vi "HFRR ADV v06 new software.vi"() -> ()   [LabVIEW 2025] (continued)
                    n2725 = Concatenate Strings(w3588, ".txt" ("string")) -> (w3589:string)
                  }
                }
                n2726 = local read "Test Date"() -> (w3580:string)
                n2727 = local read "String 45"() -> (w3494:string)
                n2728 = local read "String 31"() -> (w3579:string)
                n2729 = local read "String 32"() -> (w3578:string)
                n2730 = local read "TITTLE"() -> (w3502:string)
                n2731 = Number To Fractional String(number=w3549, width (-)=i16 6, precision (6)=i16 2) -> (F-format string=w3548:string)  [unwired: 1 in]
                n2732 = Number To Fractional String(number=w3563, width (-)=i16 6, precision (6)=i16 2) -> (F-format string=w3569:string)  [unwired: 1 in]
                n2733 = Number To Fractional String(number=w3564, width (-)=i16 6, precision (6)=i16 2) -> (F-format string=w3562:string)  [unwired: 1 in]
                n2734 = Number To Fractional String(number=w3568, width (-)=i16 6, precision (6)=i16 2) -> (F-format string=w3567:string)  [unwired: 1 in]
                n2735 = Number To Fractional String(number=w3560, width (-)=i16 6, precision (6)=i16 2) -> (F-format string=w3558:string)  [unwired: 1 in]
                n2736 = Number To Fractional String(number=w3561, width (-)=i16 6, precision (6)=i16 2) -> (F-format string=w3559:string)  [unwired: 1 in]
                n2737 = Number To Fractional String(number=w3572, width (-)=i16 6, precision (6)=i16 2) -> (F-format string=w3573:string)  [unwired: 1 in]
                n2738 = Number To Fractional String(number=w3576, precision (6)=i16 2) -> (F-format string=w3577:string)  [unwired: 2 in]
                n2739 = local read "s.NO"() -> (w3496:string)
                n2740 = Concatenate Strings("=" ("string"), w3502) -> (w3501:string)
                n2741 = Concatenate Strings("S.No," ("string"), "                                       Parameters" ("string")) -> (w3507:string)
                n2742 = Concatenate Strings(w3574, w3533, w3548, w3574, w3530, w3569, w3574, w3529, w3562, w3574, w3525, w3567, w3574, w3523, w3558, w3574, w3520, w3559, w3574, w3517, w3573, w3574, w3514, w3577) -> (w3536:string)
                n2743 = Concatenate Strings(w3506, "," ("string"), w3494, w3496, w3495, w3578, w3581, w3495, w3579, w3580, w3506) -> (w3504:string)
                n2744 = local read "Tested by"() -> (w3510:string)
                n2745 = local read "String 33"() -> (w3511:string)
                n2746 = Concatenate Strings("," ("string"), "                                                                             " ("string")) -> (w3499:string)
                n2747 = Concatenate Strings(w3501, w3497, w3504, w3497, w3507, w3536, w3497, w3499, w3511, w3510) -> (→"export":string)
                n2748 = String To Path(string=w3538) -> (path=w3545:path)
                n2749 = local read "export"() -> (w3540:string)
                n2750 = call <vilib>:"Write Characters To File.vi"("append to file? (new file:F)"=FALSE, "character string"=w3540, "file path (dialog if empty)"=w3545) -> ()  [unwired: 2 in, 1 out]
              }
            }
          }
          frame Enabled {
          }
        }
        n2751 = case shown="True" "OK Button 17" {
          frame False {
          }
          frame True {
            (unwired) 0  # existing file
            w3798 = "Choose a datalog file to open"  # prompt
            n2752 = local write "OK Button 17"(FALSE ("OK Button 17")) -> ()
            n2753 = local read "String"() -> (w3793:string)
            n2754 = String To Path(string=w3793) -> (path=w3794:path)
            n2755 = File Dialog(6:"*.duf" ("pattern"), 7:w3798, 11:w3794) -> (0:w3785:errorcluster, 3:w3804:path)  [unwired: 4 in, 2 out]
            n2756 = Unbundle(w3785) -> ()  [unwired: 3 out]
            n2757 = Open/Create/Replace File "Open File"(file path (use dialog)=w3804) -> (refnum out=w3796:refnum<file>)  [unwired: 5 in, 2 out]
            n2758 = Strip Path(path=w3804) -> (name=w3802:string)  [unwired: 1 out]
            n2759 = Path To String(path=w3804) -> (string=w3787:string)
            n2760 = while {
              tunnel: w3796 -> [w3808]
              i -> [w3805]
              stop <- w3806 continue-if-true
              (unwired) TRUE ("line mode (F)")
              n2761 = Read from Text File "Read File"(file (use dialog)=w3808) -> (text=w3807:string)  [unwired: 3 in, 3 out]
              n2762 = local write "Numeric 16"(w3805) -> ()
              n2763 = String Length(string=w3807) -> (length=w3810:i32)
              n2764 = Greater?(x=w3810, y=1) -> (0:w3806:bool)
            }
            n2765 = local write "String 29"(w3787) -> ()
            n2766 = Search and Replace String(input string=w3787, search string=".duf", replace string=".dgf" ("replace string (\"\")")) -> (result string=→"String Indicator 4":string)  [unwired: 5 in, 3 out]
            n2767 = Match Pattern(string=w3802, regular expression=".dwm") -> (before substring=w3786:string)  [unwired: 1 in, 3 out]
            "String Indicator" <- w3786
            n2768 = Match Pattern(string=w3787, regular expression=".dwm" ("substring (\"\")")) -> (before substring=w3788:string)  [unwired: 1 in, 3 out]
            "String Indicator 3" <- w3788
            n2769 = local write "TITTLE 2"(w3786) -> ()
            n2770 = String To Path(string=w3788) -> (path=w3795:path)
            "path" <- w3795
            n2771 = call <vilib>:"Read Characters From File.vi"("file path (dialog if empty)"=w3795, "start of read offset (chars.:0)"=60 ("start of read offset (chars.: 0)")) -> ("character string"=→"String Indicator 2":string)  [unwired: 4 in, 3 out]
          }
        }
        n2772 = call <vilib>:"Query Available Printers.vi"() -> ("system configured printers"=w3487:string[])  [unwired: 9 in, 2 out]
        "System Configured Printers 2" <- w3487
        n2773 = local read "OK Button 16"() -> (w3484:bool)
        n2774 = case shown="True" "OK Button 16" {
          frame False {
          }
          frame True {
            n2775 = stacked-sequence {
              frame #0 {
                n2776 = local read "Numeric 16"() -> (w3812:i32)
                n2777 = local write "Numeric 10"(w3812) -> ()
              }
              frame #1 {
                n2778 = local read "S.NO"() -> (→"s.NO":string)
                n2779 = local read "String 29"() -> (w3816:string)
                n2780 = String To Path(string=w3816) -> (path=w3815:path)
                n2781 = Open/Create/Replace File "Open File"(file path (use dialog)=w3815) -> (refnum out=w3817:refnum<file>)  [unwired: 5 in, 2 out]
                n2782 = for {
                  N: 16 -> [_]
                  tunnel: w3817 -> [w3824]
                  i -> [w3820]
                  (unwired) TRUE ("line mode (F)")
                  n2783 = Read from Text File "Read File"(file (use dialog)=w3824) -> (text=w3818:string)  [unwired: 3 in, 3 out]
                  n2784 = Match Pattern(string=w3818, regular expression="(") -> (after substring=w3823:string)  [unwired: 1 in, 3 out]
                  n2785 = Match Pattern(string=w3823, regular expression=")") -> (before substring=w3819:string)  [unwired: 1 in, 3 out]
                  n2786 = case shown="1" w3820 {
                    tunnel: w3819 -> [w3825 w3826 _ _ w3827 w3828 w3829 w3831 w3833 w3835 w3837 w3839 w3841 w3843 _]
                    tunnel: w3818 -> [_ _ _ _ _ _ _ _ _ _ _ _ _ _ _]
                    frame 0 {
                      "TITTLE" <- w3825
                    }
                    frame 1 {
                      "Sample ID" <- w3826
                    }
                    frame 2 {
                    }
                    frame 3 {
                    }
                    frame 4 {
                      "Test Date" <- w3827
                    }
                    frame 5 {
                      "Tested by" <- w3828
                    }
                    frame 6 {
                      n2787 = Fract/Exp String To Number(string=w3829) -> (number=→"Humidity before test 2":dbl)  [unwired: 3 in, 1 out]
                    }
                    frame 7 {
                      n2788 = Fract/Exp String To Number(string=w3831) -> (number=→"Temperature before test 2":dbl)  [unwired: 3 in, 1 out]
                    }
                    frame 8 {
                      n2789 = Fract/Exp String To Number(string=w3833) -> (number=→"Humidity after test 2":dbl)  [unwired: 3 in, 1 out]
                    }
                    frame 9 {
                      n2790 = Fract/Exp String To Number(string=w3835) -> (number=→"Temperature after test 2":dbl)  [unwired: 3 in, 1 out]
                    }
                    frame 10 {
                      n2791 = Fract/Exp String To Number(string=w3837) -> (number=→"MWSD 2":dbl)  [unwired: 3 in, 1 out]
                    }
                    frame 11 {
                      n2792 = Fract/Exp String To Number(string=w3839) -> (number=→"AVP 2":dbl)  [unwired: 3 in, 1 out]
                    }
                    frame 12 {
                      n2793 = Fract/Exp String To Number(string=w3841) -> (number=→"HCF 2":dbl)  [unwired: 3 in, 1 out]
                    }
                    frame 13 {
                      n2794 = Fract/Exp String To Number(string=w3843) -> (number=→"WS1.4 2":dbl)  [unwired: 3 in, 1 out]
                    }
                    frame 14, Default {
                    }
                  }
                }
              }
              frame #2 {
              }
            }
            n2795 = local write "OK Button 16"(FALSE ("OK Button 13")) -> ()
          }
        }
        n2796 = Index Array(array=w3487, index="Select Printer 3") -> (element=w3489:string)
        "Selected Printer" <- w3489
        n2797 = case shown="True" w3484 {
          frame False {
          }
          frame True {
            n2798 = flat-sequence {
              frame #0 {
              }
              frame #1 {
                n2799 = Wait (ms)(milliseconds to wait=u32 100) -> ()  [unwired: 1 out]
              }
              frame #2 {
                n2800 = local write "OK Button 16"(FALSE ("Print 3")) -> ()
              }
            }
          }
        }
        n2801 = case shown="True" "Print" {
          tunnel: w3489 -> [_ w3781]
          frame False {
          }
          frame True {
            (unwired) i16 6 ("width (-)")
            (unwired) "TESTED BY : "
            (unwired) "TESTED DATE :"
            (unwired) "SAMPLE ID : "
            (unwired) "SAMPLE DESIGN : "
            w3739 = "\r"
            w3756 = "\r"
            # "add image"
            n2802 = local read "Sample ID"() -> (w3729:string)
            n2803 = local read "Tested by"() -> (w3732:string)
            n2804 = local read "String 34"() -> (w3719:string)
            n2805 = local read "String 45"() -> (w3699:string)
            n2806 = local read "String 35"() -> (w3714:string)
            n2807 = local read "String 37"() -> (w3712:string)
            n2808 = local read "String 32"() -> (w3734:string)
            n2809 = local read "String 36"() -> (w3709:string)
            n2810 = local read "String 31"() -> (w3733:string)
            n2811 = local read "Test Date"() -> (w3730:string)
            n2812 = local read "String 33"() -> (w3735:string)
            n2813 = local read "String 38"() -> (w3705:string)
            n2814 = local read "String 39"() -> (w3702:string)
            n2815 = local write "Print"(FALSE ("Print FF")) -> ()
            n2816 = local read "S 39"() -> (w3717:string)
            n2817 = local read "S 38"() -> (w3724:string)
            n2818 = local read "Temperature before test 2"() -> (w3755:dbl)
            n2819 = local read "Temperature after test 2"() -> (w3745:dbl)
            n2820 = local read "Humidity before test 2"() -> (w3770:dbl)
            n2821 = local read "Humidity after test 2"() -> (w3754:dbl)
            n2822 = local read "MWSD 2"() -> (w3759:dbl)
            n2823 = local read "WS1.4 2"() -> (w3737:dbl)
            n2824 = Concatenate Strings("2)" ("string"), w3719) -> (w3720:string)
            n2825 = Concatenate Strings("3)" ("string"), w3717) -> (w3718:string)
            n2826 = Concatenate Strings("1)" ("string"), w3724) -> (w3723:string)
            n2827 = Concatenate Strings("4)" ("string"), w3714) -> (w3715:string)
            n2828 = Concatenate Strings("5)" ("string"), w3712) -> (w3711:string)
            n2829 = Concatenate Strings("6)" ("string"), w3709) -> (w3708:string)
            n2830 = Concatenate Strings("7)" ("string"), w3705) -> (w3706:string)
            n2831 = Concatenate Strings("8)" ("string"), w3702) -> (w3703:string)
            n2832 = local read "HCF 2"() -> (w3741:dbl)
            n2833 = local read "AVP 2"() -> (w3758:dbl)
            n2834 = local read "s.NO"() -> (w3700:string)
            n2835 = call <vilib>:"New Report.vi"("report type"=enum16{"Standard Report", "HTML"}."Standard Report") -> ("report out"=w3779:refnum<class "NI_report.lvclass">, "error out"=w3778:errorcluster)  [unwired: 13 in]
            n2836 = local read "TITTLE"() -> (w3731:string)
            n2837 = Concatenate Strings(w3756, w3699, w3700, w3756, w3734, w3729, w3756, w3733, w3730, w3756, w3735, w3732, w3756) -> (w3749:string)
            "test by" <- w3749
            n2838 = Number To Fractional String(number=w3755, width (-)=i16 6, precision (6)=i16 2) -> (F-format string=w3744:string)  [unwired: 1 in]
            n2839 = Number To Fractional String(number=w3754, width (-)=i16 6, precision (6)=i16 2) -> (F-format string=w3757:string)  [unwired: 1 in]
            n2840 = Number To Fractional String(number=w3770, width (-)=i16 6, precision (6)=i16 2) -> (F-format string=w3775:string)  [unwired: 1 in]
            n2841 = Number To Fractional String(number=w3759, width (-)=i16 6, precision (6)=i16 2) -> (F-format string=w3761:string)  [unwired: 1 in]
            n2842 = Number To Fractional String(number=w3745, width (-)=i16 6, precision (6)=i16 2) -> (F-format string=w3746:string)  [unwired: 1 in]
            n2843 = Number To Fractional String(number=w3758, width (-)=i16 6, precision (6)=i16 2) -> (F-format string=w3760:string)  [unwired: 1 in]
            n2844 = Number To Fractional String(number=w3741, width (-)=i16 6, precision (6)=i16 2) -> (F-format string=w3740:string)  [unwired: 1 in]
            n2845 = Number To Fractional String(number=w3737, precision (6)=i16 2) -> (F-format string=w3736:string)  [unwired: 2 in]
            n2846 = call-dynamic "Set Report Header Text.vi"("report in"=w3779, "center header text"=w3731, "error in (no error)"=w3778) -> ("report out"=w3750:refnum<class "NI_report.lvclass">, "error out"=w3751:errorcluster)  [unwired: 11 in]
            n2847 = Concatenate Strings(w3739, w3723, w3775, w3739, w3720, w3744, w3739, w3718, w3757, w3739, w3715, w3746, w3739, w3711, w3761, w3739, w3708, w3760, w3739, w3706, w3740, w3739, w3703, w3736) -> (w3727:string)
            "export 2" <- w3727
            n2848 = call-poly <vilib>:"Append Report Text.vi"("report in"=w3750, "text"=w3749, "error in (no error)"=w3751) -> ("report out"=w3753:refnum<class "NI_report.lvclass">, "error out"=w3752:errorcluster)  [unwired: 9 in, 2 out]
            n2849 = local read "test by"() -> (w3726:string)
            n2850 = local read "TITTLE"() -> (w3728:string)
            n2851 = call-poly <vilib>:"Append Report Text.vi"("report in"=w3753, "error in (no error)"=w3752) -> ("report out"=w3774:refnum<class "NI_report.lvclass">, "error out"=w3772:errorcluster)  [unwired: 10 in, 2 out]
            n2852 = Concatenate Strings(w3728, w3727, w3726) -> (→"output":string)
            n2853 = call-poly <vilib>:"Append Report Text.vi"("report in"=w3774, "text"=w3727, "error in (no error)"=w3772) -> ("report out"=w3773:refnum<class "NI_report.lvclass">, "error out"=w3771:errorcluster)  [unwired: 9 in, 2 out]
            n2854 = call-dynamic "Print Report.vi"("report in"=w3773, "printer name (default)"=w3781, "error in (no error)"=w3771) -> ("report out"=w3783:refnum<class "NI_report.lvclass">, "error out"=w3784:errorcluster)  [unwired: 11 in]
            n2855 = call-dynamic "Dispose Report.vi"("report in"=w3783, "error in (no error)"=w3784) -> ()  [unwired: 13 in, 1 out]
          }
        }
        n2856 = case shown="True" "Print 2" {
          frame False {
          }
          frame True {
            n2857 = flat-sequence {
              frame #0 {
                n2858 = local read "s.NO"() -> (→"s.NO 2":string)
                n2859 = Wait (ms)(milliseconds to wait=u32 20) -> ()  [unwired: 1 out]
                n2860 = local read "Sample ID  3"() -> (→"Sample ID  6":string)
                n2861 = local read "Sample ID  4"() -> (→"Sample ID  7":string)
                n2862 = local read "Sample ID"() -> (→"Sample ID  2":string)
                n2863 = local read "Tested by"() -> (→"Tested by 2":string)
                n2864 = local read "Test Date"() -> (→"Test Date 2":string)
                n2865 = local read "Humidity after test 3"() -> (→"Humidity after test 4":dbl)
                n2866 = local read "Ref A Test Date :"() -> (→"TITTLE 4":string)
                n2867 = local read "Temperature before test 3"() -> (w3606:dbl)
                n2868 = local read "Temperature before test 3"() -> (→"Temperature after test 5":dbl)
                n2869 = local read "Temperature after test 3"() -> (→"Temperature after test 4":dbl)
                n2870 = local read "Humidity before test 3"() -> (→"Humidity before test 4":dbl)
                n2871 = local write "Temperature before test 3"(w3606) -> ()
                n2872 = local read "image data"() -> (w3597:T11)
                n2873 = String To Path(string="C:\\LAB-IQ\\im\\Temp_resized.jpg") -> (path=w3598:path)
                "path 2" <- w3598
                n2874 = call <vilib>:"Write JPEG File.vi"("image data"=w3597, "path to JPEG file"=w3598) -> ()  [unwired: 8 in, 2 out]
                "Ref A Test Date :" <- "Ref A Test Date :"
                "Ref B Test Date :" <- "Ref B Test Date :"
                "Ref B Scar Value :" <- "Ref B Scar Value :"
                "Ref A Scar Value :" <- "Ref A Scar Value :"
              }
              frame #1 {
                (unwired) HTML_Report_Image_Alignment."MIDDLE" ("alignment (default)")
                w3634 = u16 0 items=["portrait", "landscape"] ("orientation (portrait)")
                (unwired) HTML_Report_Image_Alignment."ABSMIDDLE" ("alignment (default)")
                (unwired) "TESTED BY : "
                (unwired) "TESTED DATE :"
                (unwired) "SAMPLE ID : "
                (unwired) "SAMPLE DESIGN : "
                w3667 = "\r"
                # "add image"
                n2875 = Wait (ms)(milliseconds to wait=u32 20) -> ()  [unwired: 1 out]
                n2876 = local read "Sample ID  2"() -> (w3660:string)
                n2877 = local read "Wear Scar X"() -> (w3632:dbl)
                "Length ( microns ) 2" <- w3632
                n2878 = local read "Wear Scar Y"() -> (w3631:dbl)
                "Wear Scar Y ( microns ) :" <- w3631
                n2879 = local read "Test Date 2"() -> (w3661:string)
                n2880 = local read "Tested by 2"() -> (w3662:string)
                n2881 = local read "String 46"() -> (w3658:string)
                n2882 = local read "String 48"() -> (w3664:string)
                n2883 = local read "String 47"() -> (w3663:string)
                n2884 = local read "String 49"() -> (w3665:string)
                n2885 = local read "String 10"() -> (w3618:string)
                n2886 = local read "s.NO 2"() -> (w3659:string)
                n2887 = Add(x=w3632, y=w3631) -> (x+y=w3630:dbl)
                n2888 = call <vilib>:"New Report.vi"("report type"=enum16{"Standard Report", "HTML"}."HTML") -> ("report out"=w3638:refnum<class "NI_report.lvclass">, "error out"=w3636:errorcluster)  [unwired: 13 in]
                n2889 = Concatenate Strings(w3667, w3658, w3659, w3667, w3664, w3660, w3667, w3663, w3661, w3667, w3665, w3662, w3667) -> (→"test by 2":string)
                n2890 = Concatenate Strings("C:\\LAB-IQ\\Data\\" ("string"), w3618, ".jpg" ("string")) -> ()  [unwired: 1 out]
                n2891 = Divide(x=w3630, y=2.0) -> (x/y=→"Mean Wear ( microns) :":dbl)
                n2892 = call-dynamic "Set Report Orientation.vi"("report in"=w3638, "orientation (portrait)"=w3634, "error in (no error)"=w3636) -> ("report out"=w3637:refnum<class "NI_report.lvclass">, "error out"=w3635:errorcluster)  [unwired: 11 in]
                n2893 = for {
                  N: 5 -> [_]
                  tunnel: w3637 -> [w3688]
                  tunnel: [w3687] -> w3616
                  tunnel: w3635 -> [w3686]
                  tunnel: [w3685] -> w3615
                  n2894 = call-dynamic "Set Report Tab Width.vi"("report in"=w3688, "error in (no error)"=w3686) -> ("report out"=w3687:refnum<class "NI_report.lvclass">, "error out"=w3685:errorcluster)  [unwired: 12 in]
                }
                n2895 = local read "TITTLE"() -> (w3633:string)
                n2896 = call-dynamic "Set Report Header Text.vi"("report in"=w3616, "center header text"=w3633, "error in (no error)"=w3615) -> ("report out"=w3654:refnum<class "NI_report.lvclass">, "error out"=w3653:errorcluster)  [unwired: 11 in]
                n2897 = for {
                  N: 1 -> [_]
                  tunnel: [w3692] -> w3640
                  tunnel: [w3691] -> w3639
                  tunnel: w3654 -> [w3690]
                  tunnel: w3653 -> [w3689]
                  n2898 = call-dynamic "New Report Line.vi"("report in"=w3690, "error in (no error)"=w3689) -> ("report out"=w3692:refnum<class "NI_report.lvclass">, "error out"=w3691:errorcluster)  [unwired: 12 in]
                }
                n2899 = for {
                  N: 2 -> [_]
                  tunnel: [w3684] -> w3646
                  tunnel: [w3683] -> w3645
                  tunnel: w3640 -> [w3682]
                  tunnel: w3639 -> [w3681]
                  n2900 = call-dynamic "New Report Line.vi"("report in"=w3682, "error in (no error)"=w3681) -> ("report out"=w3684:refnum<class "NI_report.lvclass">, "error out"=w3683:errorcluster)  [unwired: 12 in]
                }
                n2901 = for {
                  N: 25 -> [_]
                  tunnel: w3646 -> [w3680]
                  tunnel: w3645 -> [w3678]
                  tunnel: [w3679] -> w3649
                  tunnel: [w3677] -> w3648
                  n2902 = call-dynamic "Set Report Tab Width.vi"("report in"=w3680, "error in (no error)"=w3678) -> ("report out"=w3679:refnum<class "NI_report.lvclass">, "error out"=w3677:errorcluster)  [unwired: 12 in]
                }
                n2903 = control-ref of="Tab Control 9"() -> (w3644:refnum<vi>)
                n2904 = call-dynamic "Append Control Image to Report.vi"("report in"=w3649, "alignment (default)"=HTML_Report_Image_Alignment."ABSMIDDLE", "ctrl reference"=w3644, "error in (no error)"=w3648) -> ("report out"=w3643:refnum<class "NI_report.lvclass">, "error out"=w3642:errorcluster)  [unwired: 8 in, 2 out]
                n2905 = for {
                  N: 3 -> [_]
                  tunnel: [w3676] -> w3627
                  tunnel: [w3675] -> w3626
                  tunnel: w3643 -> [w3674]
                  tunnel: w3642 -> [w3673]
                  n2906 = call-dynamic "New Report Line.vi"("report in"=w3674, "error in (no error)"=w3673) -> ("report out"=w3676:refnum<class "NI_report.lvclass">, "error out"=w3675:errorcluster)  [unwired: 12 in]
                }
                n2907 = for {
                  N: 100 -> [_]
                  tunnel: w3627 -> [w3672]
                  tunnel: w3626 -> [w3670]
                  tunnel: [w3671] -> w3623
                  tunnel: [w3669] -> w3621
                  n2908 = call-dynamic "Set Report Tab Width.vi"("report in"=w3672, "error in (no error)"=w3670) -> ("report out"=w3671:refnum<class "NI_report.lvclass">, "error out"=w3669:errorcluster)  [unwired: 12 in]
                }
                n2909 = String To Path(string="C:\\LAB-IQ\\im\\Temp_resized.jpg") -> (path=w3613:path)
                n2910 = call-poly <vilib>:"Append Image to Report.vi"("report in"=w3623, "path or URL of image"=w3613, "error in (no error)"=w3621) -> ("report out"=w3622:refnum<class "NI_report.lvclass">, "error out"=w3620:errorcluster)  [unwired: 9 in, 2 out]
                n2911 = call-poly <vilib>:"Open HTML Report in Browser.vi"("report in"=w3622, "error in (no error)"=w3620) -> ("report out"=w3657:refnum<class "NI_report.lvclass">, "error out"=w3656:errorcluster)  [unwired: 11 in, 1 out]
                n2912 = call-dynamic "Dispose Report.vi"("report in"=w3657, "error in (no error)"=w3656) -> ()  [unwired: 13 in, 1 out]
              }
              frame #2 {
              }
              frame #3 {
                n2913 = disable-structure shown="Disabled" {
                  frame Disabled {
                    n2914 = local read "String 10"() -> (w3697:string)
                    n2915 = Concatenate Strings("C:\\LAB-IQ-NXT\\Data\\" ("string"), w3697, ".jpg" ("string")) -> (w3695:string)
                    n2916 = String To Path(string=w3695) -> (path=w3694:path)
                    n2917 = Delete(path (use dialog)=w3694) -> ()  [unwired: 4 in, 3 out]
                  }
                  frame Enabled {
                  }
                }
                n2918 = local write "Print 2"(FALSE ("Print")) -> ()
              }
            }
          }
        }
      }
    }
    n2919 = property on="SetTemp" class="DigNum (strict)"("Disabled"=w1640) -> ()  [unwired: 2 in, 2 out]
    n2920 = Multiply(x=w1630, y=w1632) -> (x*y=w1631:dbl)
    n2921 = local read "MWSD"() -> (w1629:dbl)
    n2922 = Add(x=w1631, y=w1629) -> (x+y=→"WS1.4":dbl)
    n2923 = Wait (ms)(milliseconds to wait=u32 50) -> ()  [unwired: 1 out]
    n2924 = Wait (ms)(milliseconds to wait=u32 50) -> ()  [unwired: 1 out]
    n2925 = local read "Quit"() -> (w1628:bool)
  }
  n2926 = VISA Close(VISA resource name=w52, error in (no error)=w51) -> (error out=w49:errorcluster)
  n2927 = call <vilib>:"Clear Errors.vi"("error in (no error)"=w49) -> ()  [unwired: 5 in, 2 out]
  n2928 = VISA Close(VISA resource name=w37, error in (no error)=w36) -> ()  [unwired: 1 out]
  n2929 = while {
    tunnel: [w3856] -> w46
    shift-right: [w3849] -> _
    shift-left: 0.0 -> [w3852]
    shift-right: [w3848] -> _
    shift-left: 0.0 -> [w3851]
    shift-right: [w3847] -> _
    shift-left: 400.0 ("vc_cmd") -> [w3850]
    stop <- w3856 stop-if-true
    # "PID LOGIC"
    n2930 = local read "RUN"() -> (w3854:bool)
    n2931 = local read "Auto Start Test"() -> (w3853:bool)
    n2932 = local read "START TEMP"() -> (w3845:bool)
    n2933 = Or(x=w3854, y=w3853) -> (x .or. y?=w3855:bool)
    n2934 = And(x=w3855, y=w3845) -> (x .and. y?=w3846:bool)
    n2935 = Wait (ms)(milliseconds to wait=u32 20) -> ()  [unwired: 1 out]
    n2936 = case shown="True" w3846 {
      tunnel: [400.0 ("out_vc_cmd") w3876] -> w3847
      tunnel: [w3859 w3878] -> w3848
      tunnel: [w3859 w3877] -> w3849
      tunnel: w3852 -> [_ w3867]
      tunnel: w3851 -> [_ w3866]
      tunnel: w3850 -> [_ w3865]
      frame False {
        w3859 = 0.0 ("error_out")
      }
      frame True {
        n2937 = local read "Set Strk"() -> (w3862:dbl)
        n2938 = local read "LVDT STROKE"() -> (w3860:dbl)
        n2939 = Add(x=w3862, y="Add up Stroke") -> (x+y=w3863:dbl)
        n2940 = formula code="// Zero-Hardcode Explicit Positional-Form PID Engine\n// Inputs: target_stroke, measured_stroke, dt, prev_error, integral_accumulator_in, prev_vc_cmd\n//         kp, ki, kd, max_step_change, max_amplitude, min_amplitude, startup_cmd\n// Outputs: vc_cmd, error_out, out_error, integral_accumulator_out, out_vc_cmd\n\n// 1. Calculate Tracking Error\nfloat current_error = target_stroke - measured_stroke;\nerror_out = current_error;\n\n// 2. Compute Proportional Term\nfloat p_term = kp * current_error;\n\n// 3. Compute Derivative Term\nfloat d_term = 0.0;\nif (dt > 0.0) {\n    d_term = kd * ((current_error - prev_error) / dt);\n}\n\n// 4. Update and Accumulate Integral Term\nfloat current_integral = integral_accumulator_in + (current_error * dt);\nfloat i_term = ki * current_integral;\n\n// 5. Calculate Ideal Target Command\nfloat ideal_command = startup_cmd + p_term + i_term + d_term;\n\n// 6. Anti-Windup Protection (Back-calculation method)\nif (ideal_command > max_amplitude) {\n    float excess = ideal_command - max_amplitude;\n    if (ki > 0.0) {\n        current_integral -= excess / ki;\n    }\n    ideal_command = max_amplitude;\n} else if (ideal_command < min_amplitude) {\n    float excess = ideal_command - min_amplitude;\n    if (ki > 0.0) {\n        current_integral -= excess / ki;\n    }\n    ideal_command = min_amplitude;\n}\n\n// 7. Apply Loop Rate Limiting (Protects voice coil from large voltage steps)\nfloat raw_adjustment = ideal_command - prev_vc_cmd;\n\nif (raw_adjustment > max_step_change) {\n    raw_adjustment = max_step_change;\n} else if (raw_adjustment < -max_step_change) {\n    raw_adjustment = -max_step_change;\n}\n\nfloat next_vc_cmd = prev_vc_cmd + raw_adjustment;\n\n// Final Output Safety Safeguard Clamping\nif (next_vc_cmd > max_amplitude) {\n    next_vc_cmd = max_amplitude;\n} else if (next_vc_cmd < min_amplitude) {\n    next_vc_cmd = min_amplitude;\n}\n\n// 8. Map to Shift Registers for memory persistence\nvc_cmd = next_vc_cmd;\nout_error = current_error;                     \nintegral_accumulator_out = current_integral;  \nout_vc_cmd = next_vc_cmd;"("target_stroke"=w3863, "measured_stroke"=w3860, "dt"="dt", "integral_accumulator_in"=w3866, "prev_error"=w3867, "prev_vc_cmd"=w3865, "kp"="kp", "ki"="ki", "kd"="kd", "max_step_change"="max_step_change", "max_amplitude"="max_amplitude", "min_amplitude"="min_amplitude", "startup_cmd"="startup_cmd") -> ("vc_cmd"=w3882:dbl, "out_error"=w3877:dbl, "integral_accumulator_out"=w3878:dbl, "out_vc_cmd"=w3876:dbl)  [unwired: 1 out]
        "output Vpp" <- w3882
        n2941 = Number To Fractional String(number=w3882, precision (6)=i16 1) -> (F-format string=w3880:string)  [unwired: 2 in]
        n2942 = Concatenate Strings("DAC;" ("string"), w3880) -> (w3864:string)
        n2943 = local write "Command"(w3864) -> ()
        "prev_error" <- w3867
        "integral_accumulator_in" <- w3866
        "prev_vc_cmd" <- w3865
      }
    }
    n2944 = local read "Quit"() -> (w3856:bool)
  }
  n2945 = Or(x=w42, y=w41) -> (x .or. y?=w43:bool)
  n2946 = Or(x=w39, y=w43) -> (x .or. y?=w48:bool)
  n2947 = control-ref of="new picture"() -> ()  [unwired: 1 out]
  n2948 = Or(x=w54, y=w48) -> (x .or. y?=w45:bool)
  n2949 = Or(x=w45, y=w46) -> (x .or. y?=w40:bool)
  n2950 = while {
    tunnel: [w3883] -> w53
    i -> [w3890]
    stop <- w3883 stop-if-true
    n2951 = local read "Quit"() -> (w3883:bool)
    n2952 = Equal To 0?(x=w3890) -> (x = 0?=w3888:bool)
    n2953 = call "Elapsed Time3"("Time Target (s)"=45.0, "Auto Reset"=TRUE) -> ("Time has Elapsed"=w3887:bool)  [unwired: 10 in, 7 out]
    n2954 = Wait (ms)(milliseconds to wait=u32 50) -> ()  [unwired: 1 out]
    n2955 = Or(x=w3887, y=w3888) -> (x .or. y?=w3889:bool)
    n2956 = case shown="True" w3889 {
      frame False {
      }
      frame True {
        n2957 = call <vilib>:"System Exec.vi"("run minimized? (F)"=TRUE, "error in (no error)"="error in (no error)", "command line"="powercfg.exe -change -monitor-timeout-ac 0") -> ("error out"=w3901:errorcluster)  [unwired: 5 in, 3 out]
        n2958 = call <vilib>:"System Exec.vi"("run minimized? (F)"=TRUE, "error in (no error)"=w3901, "command line"="powercfg.exe -change -disk-timeout-ac 0") -> ("error out"=w3900:errorcluster)  [unwired: 5 in, 3 out]
        n2959 = call <vilib>:"System Exec.vi"("run minimized? (F)"=TRUE, "error in (no error)"=w3900, "command line"="powercfg.exe -change -standby-timeout-ac 0") -> ("error out"=w3899:errorcluster)  [unwired: 5 in, 3 out]
        n2960 = call <vilib>:"System Exec.vi"("run minimized? (F)"=TRUE, "error in (no error)"=w3899, "command line"="powercfg.exe -change -hibernate-timeout-ac 0") -> ("error out"=w3898:errorcluster)  [unwired: 5 in, 3 out]
        n2961 = call <vilib>:"Simple Error Handler.vi"("error in (no error)"=w3898) -> ("error out"=w3904:errorcluster)  [unwired: 4 in, 4 out]
        n2962 = call <vilib>:"Clear Errors.vi"("error in (no error)"=w3904) -> ("error out"=→"error out":errorcluster)  [unwired: 5 in, 1 out]
      }
    }
  }
  n2963 = Compound Arithmetic op=OR(w56, w40, w53) -> (w55:bool)
  n2964 = flat-sequence {
    tunnel: w55 -> [_]
    tunnel: [w3906] -> w18
    tunnel: w18 -> [_]
    frame #0 {
      n2965 = call "CLOSE CONNECTION.vi"() -> ("error out"=w3906:errorcluster)  [unwired: 11 in]
    }
    frame #1 {
      n2966 = Quit LabVIEW(quit? (T)=TRUE) -> ()
      n2967 = local write "Quit"(FALSE ("EXIT")) -> ()
    }
  }
  n2968 = property on="Heater Button" class="Bool (strict)"("Visible"=TRUE) -> ()  [unwired: 2 in, 2 out]
  n2969 = disable-structure shown="Disabled" {
    disable-tunnel: _ -> [w3912 _]
    disable-tunnel: _ -> [w3909 _]
    disable-tunnel: _ -> [w3910 _]
    frame Disabled {
      n2970 = disable-structure shown="Disabled" {
        disable-tunnel: [w3919 _] -> w3911
        frame Disabled {
          n2971 = while {
            shift-right: [w3961] -> w3917
            shift-left: errorcluster {"status"=TRUE, "code"=0, "source"="Init"} ("error out") -> [w3926]
            shift-right: [w3960] -> w3916
            shift-left: _ -> [w3927]
            shift-right: [w3959] -> _
            shift-left: "" -> [w3958]
            tunnel: [w3920] -> w3919
            shift-right: ["Set Rh"] -> _
            shift-left: 0.0 ("Set Rh") -> [w3952]
            tunnel: [w3929] -> _
            i -> [w3929]
            stop <- w3920 stop-if-true
            n2972 = flat-sequence {
              tunnel: w3926 -> [w3964]
              tunnel: [w3964] -> w3925
              frame #0 {
                n2973 = Wait (ms)(milliseconds to wait=u32 200) -> ()  [unwired: 1 out]
              }
            }
            n2974 = local read "Com Port 3"() -> (w3928:refnum<visa-resource-name>)
            n2975 = local read "Humidity Str Rec"() -> (w3930:string)
            n2976 = Not Equal?(x="Set Rh", y=w3952) -> (x != y?=w3957:bool)
            n2977 = Number To Decimal String(number="Set Rh") -> (decimal integer string=w3955:string)  [unwired: 1 in]
            n2978 = Not Equal?(x=w3928, y=w3927) -> (x != y?=w3923:bool)
            n2979 = Concatenate Strings("#setPoint00" ("string"), w3955) -> (w3956:string)
            n2980 = case shown="False" w3957 {
              tunnel: w3956 -> [_ w3976]
              frame False {
                n2981 = local read "Humidity"() -> (w3973:bool)
                n2982 = case shown="True" w3973 {
                  frame False {
                    n2983 = local write "Humidity Str Send"("stop" ("Humidity Str Send")) -> ()
                  }
                  frame True {
                    n2984 = local write "Humidity Str Send"("start" ("Humidity Str Send")) -> ()
                  }
                }
              }
              frame True {
                n2985 = local write "Humidity Str Send"(w3976) -> ()
              }
            }
            n2986 = Or(x=w3923) -> (y=w3921:bool, x .or. y?=w3922:bool)
            n2987 = String Subset(string=w3930, offset (0)=7) -> (substring=w3945:string)  [unwired: 1 in]
            n2988 = Match Pattern(string=w3930, regular expression="?") -> (offset past match=w3948:i32)  [unwired: 1 in, 3 out]
            n2989 = Match Pattern(string=w3930, regular expression="v") -> (offset past match=w3951:i32)  [unwired: 1 in, 3 out]
            n2990 = case shown="True" w3922 {
              tunnel: w3925 -> [w3962 _]
              tunnel: [w3962 errorcluster {"status"=TRUE, "code"=0, "source"="Init"} ("error out")] -> w3924
              frame False {
              }
              frame True {
              }
            }
            n2991 = Equal?(x=w3948, y=-1) -> (x = y?=w3932:bool)
            n2992 = Match Pattern(string=w3945, regular expression="g") -> (after substring=w3946:string, offset past match=w3937:i32)  [unwired: 1 in, 2 out]
            n2993 = Match Pattern(string=w3945, regular expression="y") -> (after substring=w3944:string, offset past match=w3938:i32)  [unwired: 1 in, 2 out]
            n2994 = Greater?(x=w3938, y=w3937) -> (0:w3943:bool)
            n2995 = Greater Or Equal To 0?(x=w3938) -> (x >= 0?=w3935:bool)
            n2996 = Greater Or Equal To 0?(x=w3937) -> (x >= 0?=w3936:bool)
            n2997 = Or(x=w3935, y=w3936) -> (x .or. y?=w3934:bool)
            n2998 = Greater Or Equal To 0?(x=w3951) -> (x >= 0?=w3933:bool)
            n2999 = Select(t=w3944, s=w3943, f=w3946) -> (s? t:f=w3939:string)
            n3000 = case shown="Error" w3924 {
              selector: w3924 -> [w3989 w4035]
              tunnel: [w3987 w4028] -> w3961
              tunnel: w3927 -> [w3990 w4034]
              tunnel: [w3988 w4037] -> w3960
              tunnel: w3958 -> [w3977 w4036]
              tunnel: [w3984 w4036] -> w3959
              frame No Error {
                n3001 = call "Elapsed Time7"() -> ("Time has Elapsed"=w3983:bool)  [unwired: 12 in, 7 out]
                n3002 = Not Equal?(x="Humidity Str Send", y=w3977) -> (x != y?=w3979:bool)
                n3003 = Or(x=w3979, y=w3983) -> (x .or. y?=w3982:bool)
                n3004 = Select(t="Humidity Str Send", s=w3979, f="vals" ("regular expression")) -> (s? t:f=w3978:string)
                n3005 = Or(x=w3982, y="Send") -> (x .or. y?=w3986:bool)
                n3006 = case shown="True" w3986 {
                  tunnel: [w3993 w3998] -> w3987
                  tunnel: w3990 -> [w3992 w4006]
                  tunnel: w3989 -> [w3993 w4005]
                  tunnel: [w3992 w3999] -> w3988
                  tunnel: w3978 -> [_ w4004]
                  tunnel: [w3991 w3995] -> w3984
                  tunnel: "Humidity Str Send" -> [_ w3996]
                  tunnel: w3979 -> [_ w3997]
                  tunnel: w3977 -> [w3991 w3994]
                  frame False {
                  }
                  frame True {
                    n3007 = flat-sequence {
                      tunnel: w4006 -> [w4014]
                      tunnel: w4005 -> [w4013]
                      tunnel: w4004 -> [w4010]
                      tunnel: [w4012] -> w4003
                      tunnel: [w4011] -> w4002
                      tunnel: w4003 -> [w4017]
                      tunnel: w4002 -> [w4016]
                      tunnel: [w4017] -> w4001
                      tunnel: [w4016] -> w4000
                      tunnel: w4001 -> [w4024]
                      tunnel: w4000 -> [w4023]
                      tunnel: [w4022] -> w3999
                      tunnel: [w4021] -> w3998
                      frame #0 {
                        n3008 = local write "Ser Led"(TRUE ("Boolean 4")) -> ()
                        n3009 = Concatenate Strings(w4010, "\r") -> (w4009:string)
                        n3010 = VISA Write(VISA resource name=w4014, write buffer=w4009, error in (no error)=w4013) -> (VISA resource name out=w4012:refnum<visa-resource-name>, error out=w4011:errorcluster)  [unwired: 1 out]
                      }
                      frame #1 {
                        n3011 = Wait (ms)(milliseconds to wait="wait") -> ()  [unwired: 1 out]
                      }
                      frame #2 {
                        w4019 = FALSE ("Send")
                        n3012 = property class="Instr"(reference=w4024, error in=w4023) -> (reference out=w4025:refnum<visa-resource-name>, error out=w4026:errorcluster, "Serial Settings:Number of Bytes at Serial Port"=w4018:u32)
                        n3013 = local write "Send"(w4019) -> ()
                        n3014 = local write "Ser Led"(w4019) -> ()
                        n3015 = VISA Read(VISA resource name=w4025, byte count=w4018, error in (no error)=w4026) -> (VISA resource name out=w4022:refnum<visa-resource-name>, read buffer=→"Humidity Str Rec":string, error out=w4021:errorcluster)  [unwired: 1 out]
                      }
                    }
                    n3016 = Select(t=w3996, s=w3997, f=w3994) -> (s? t:f=w3995:string)
                  }
                }
              }
              frame Error {
                w4042 = u16 0 items=["None"=0, "XON/XOFF"=1, "RTS/CTS"=2, "DTR/DSR"=4] ("flow control")
                w4038 = u16 0 items=["None", "Odd", "Even", "Mark", "Space"] ("parity")
                w4041 = u16 10 items=["1.0"=10, "1.5"=15, "2.0"=20] ("stop bits")
                n3017 = VISA Close(VISA resource name=w4034, error in (no error)=w4035) -> (error out=w4033:errorcluster)
                n3018 = local write "humid"("" ("humid")) -> ()
                n3019 = local write "Humidity Str Rec"("" ("Humidity Str Rec")) -> ()
                n3020 = call <vilib>:"Clear Errors.vi"("error in (no error)"=w4033) -> ("error out"=w4032:errorcluster)  [unwired: 5 in, 1 out]
                n3021 = local read "Com Port 3"() -> (w4031:refnum<visa-resource-name>)
                n3022 = call-poly "VISA Configure Serial Port"("VISA resource name"=w4031, "timeout (10sec)"=u32 1000, "termination char\n(0xA = '\\n' = LF)"=u8 10 ("termination char\n(0xA = '\\n' = LF)"), "Enable Termination\nChar (T)"=FALSE ("Enable Termination Char (T)"), "data bits (8)"=u16 8 ("data bits"), "parity (0:none)"=w4038, "error in (no error)"=w4032, "stop bits (10: 1 bit)"=w4041, "flow control (0:none)"=w4042) -> ("VISA resource name out"=w4037:refnum<visa-resource-name>, "baud rate (9600)"=w4029:u32, "error out"=w4028:errorcluster)  [unwired: 4 in]
              }
            }
            n3023 = Compound Arithmetic op=AND(w3933, w3932, w3934) -> (w3931:bool)
            n3024 = case shown="True" w3931 {
              tunnel: w3930 -> [_ _]
              tunnel: w3939 -> [_ w3969]
              frame False {
              }
              frame True {
                w3967 = " " ("regular expression")
                n3025 = Match Pattern(string=w3969, regular expression=" ") -> (after substring=w3971:string)  [unwired: 1 in, 3 out]
                n3026 = Match Pattern(string=w3971, regular expression=w3967) -> (before substring=→"humid":string, after substring=w3968:string)  [unwired: 1 in, 2 out]
                n3027 = Match Pattern(string=w3968, regular expression=w3967) -> (before substring=→"temp_@Rh sensor":string)  [unwired: 1 in, 3 out]
              }
            }
            n3028 = local read "Quit"() -> (w3920:bool)
          }
          n3029 = VISA Close(VISA resource name=w3916, error in (no error)=w3917) -> (error out=w3913:errorcluster)
          n3030 = call <vilib>:"Clear Errors.vi"("error in (no error)"=w3913) -> ()  [unwired: 5 in, 2 out]
        }
        frame Enabled {
        }
      }
    }
    frame Enabled {
    }
  }
  n3031 = while {
    tunnel: [w4049] -> _
    i -> [w4049]
    stop <- w4045 stop-if-true
    # "Langauage selection"
    n3032 = Equal?(x="Lan flag", y=22.0) -> ()  [unwired: 1 out]
    n3033 = disable-structure shown="Disabled" {
      frame Disabled {
        n3034 = stacked-sequence {
          frame #0 {
            n3035 = case shown="\"Russian\"" "Language Selection" {
              tunnel: [0 1] -> w4051
              frame "English", Default {
              }
              frame "Russian" {
              }
            }
            n3036 = for {
              N: 130 -> [_]
              tunnel: "Table" -> [w4060]
              tunnel: w4051 -> [w4059]
              i -> [w4058]
              n3037 = Index Array(array=w4060, index (row)=w4058, index (col)=w4059) -> (element=w4057:string)
              n3038 = case shown="123" w4058 {
                tunnel: w4057 -> [w4061 w4062 _ w4063 w4064 w4065 w4066 w4067 w4068 w4069 w4070 w4071 w4072 w4073 w4074 w4075 w4076 w4077 w4078 w4079 w4080 w4081 w4082 w4083 w4084 w4085 w4086 w4087 w4088 _ _ w4089 w4090 w4091 w4092 w4093 w4094 w4103 w4110 w4117 w4124 w4128 w4131 w4134 w4136 w4138 w4139 w4140 w4141 w4142 w4143 w4144 w4145 w4146 w4147 w4148 w4149 w4150 w4151 w4152 w4153 w4154 w4155 w4156 w4157 w4158 w4159 w4160 w4161 w4162 w4163 w4164 w4165 w4166 w4167 w4168 w4169 w4170 w4171 w4172 w4173 w4174 w4175 w4176 w4177 w4178 w4179 w4180 w4181 w4182 w4183 w4184 w4185 w4186 w4187 w4188 w4189 w4190 w4191 w4192 w4193 w4194 w4195 w4196 w4197 _ w4198 w4199 w4200 w4201 w4202 w4203 w4204 w4205 w4206 w4207 w4208 w4209 w4210 _ w4211 w4212 w4213 w4214 w4215 w4216 _]
                frame 0 {
                  n3039 = local write "S"(w4061) -> ()
                }
                frame 1 {
                  n3040 = local write "S 2"(w4062) -> ()
                }
                frame 2 {
                }
                frame 3 {
                  n3041 = local write "S 4"(w4063) -> ()
                }
                frame 4 {
                  n3042 = property on="FILE" class="Str"("Caption.Text"=w4064) -> ()  [unwired: 2 in, 2 out]
                }
                frame 5 {
                  n3043 = property on="Fuel Discription :" class="Str"("Caption.Text"=w4065) -> ()  [unwired: 2 in, 2 out]
                }
                frame 6 {
                  n3044 = property on="Remarks :" class="Str"("Caption.Text"=w4066) -> ()  [unwired: 2 in, 2 out]
                }
                frame 7 {
                  n3045 = property on="Save & Continue" class="Bool (strict)"("Boolean Text.Text"=w4067) -> ()  [unwired: 2 in, 2 out]
                }
                frame 8 {
                }
                frame 9 {
                  n3046 = property on="Set Hz" class="DigNum (strict)"("Caption.Text"=w4069) -> ()  [unwired: 2 in, 2 out]
                }
                frame 10 {
                  "String 3" <- w4070
                }
                frame 11 {
                  n3047 = property on="NORMAL LOAD" class="DigNum (strict)"("Caption.Text"=w4071) -> ()  [unwired: 2 in, 2 out]
                }
                frame 12 {
                  "String 5" <- w4072
                }
                frame 13 {
                  n3048 = property on="Set Temp" class="DigNum (strict)"("Caption.Text"=w4073) -> ()  [unwired: 2 in, 2 out]
                }
                frame 14 {
                  n3049 = local write "S 15"(w4074) -> ()
                }
                frame 15 {
                  n3050 = property on="Set Rh" class="DigNum (strict)"("Caption.Text"=w4075) -> ()  [unwired: 2 in, 2 out]
                }
                frame 16 {
                  "String 13" <- w4076
                  "String 26" <- w4076
                }
                frame 17 {
                  n3051 = local write "S 18"(w4077) -> ()
                }
                frame 18 {
                  "String 17" <- w4078
                }
                frame 19 {
                  n3052 = property on="test time" class="DigNum (strict)"("Caption.Text"=w4079) -> ()  [unwired: 2 in, 2 out]
                }
                frame 20 {
                  "String 18" <- w4080
                  "String 22" <- w4080
                }
                frame 21 {
                  n3053 = property on="Elapsed time" class="DigNum (strict)"("Caption.Text"=w4081) -> ()  [unwired: 2 in, 2 out]
                }
                frame 22 {
                  n3054 = property on="Samplingtime 2" class="DigNum (strict)"("Caption.Text"=w4082) -> ()  [unwired: 2 in, 2 out]
                }
                frame 23 {
                  "String 21" <- w4083
                }
                frame 24 {
                  n3055 = property on="Countdown" class="DigNum (strict)"("Caption.Text"=w4084) -> ()  [unwired: 2 in, 2 out]
                }
                frame 25 {
                  n3056 = property on="Countdown 2" class="DigNum (strict)"("Caption.Text"=w4085) -> ()  [unwired: 2 in, 2 out]
                }
                frame 26 {
                  n3057 = property on="Engage" class="Bool (strict)"("Boolean Text.Text"=w4086) -> ()  [unwired: 2 in, 2 out]
                }
                frame 27 {
                  n3058 = property on="Boolean  4" class="Bool (strict)"("Boolean Text.Text"=w4087) -> ()  [unwired: 2 in, 2 out]
                }
                frame 28 {
                  n3059 = property on="Test \nStatus" class="Bool (strict)"("Boolean Text.Text"=w4088) -> ()  [unwired: 2 in, 2 out]
                }
                frame 29 {
                }
                frame 30 {
                }
                frame 31 {
                }
                frame 32 {
                  n3060 = property on="RSTCOF" class="Bool"("Boolean Text.Text"=w4090) -> ()  [unwired: 2 in, 2 out]
                  n3061 = property on="RST FF" class="Bool"("Boolean Text.Text"=w4090) -> ()  [unwired: 2 in, 2 out]
                  n3062 = property on="RST TEMP" class="Bool"("Boolean Text.Text"=w4090) -> ()  [unwired: 2 in, 2 out]
                  n3063 = property on="RSTV1 3" class="Bool"("Boolean Text.Text"=w4090) -> ()  [unwired: 2 in, 2 out]
                  n3064 = property on="rstv2" class="Bool"("Boolean Text.Text"=w4090) -> ()  [unwired: 2 in, 2 out]
                  n3065 = property on="RSTV1 2" class="Bool"("Boolean Text.Text"=w4090) -> ()  [unwired: 2 in, 2 out]
                  n3066 = property on="RST CP" class="Bool"("Boolean Text.Text"=w4090) -> ()  [unwired: 2 in, 2 out]
                }
                frame 33 {
                  "S 61" <- w4091
                }
                frame 34 {
                  "String 23" <- w4092
                }
                frame 35 {
                  n3067 = property on="Rh Before" class="DigNum (strict)"("Caption.Text"=w4093) -> ()  [unwired: 2 in, 2 out]
                }
                frame 36 {
                  n3068 = Match Pattern(string=w4094, regular expression=",") -> (before substring=→"bs":string, after substring=→"as":string)  [unwired: 1 in, 2 out]
                  n3069 = property on="Rh After" class="DigNum (strict)"("Caption.Text"=w4094) -> ()  [unwired: 2 in, 2 out]
                }
                frame 37 {
                  n3070 = Match Pattern(string=w4103, regular expression=",") -> (before substring=w4102:string, after substring=w4101:string)  [unwired: 1 in, 2 out]
                  "bs" <- w4102
                  "as" <- w4101
                  n3071 = Concatenate Strings(w4102, w4101) -> (w4098:string)
                  n3072 = property on="Humidity before test 2" class="DigNum (strict)"("Caption.Text"=w4098) -> ()  [unwired: 2 in, 2 out]
                  n3073 = property on="Humidity before test" class="DigNum (strict)"("Caption.Text"=w4098) -> ()  [unwired: 2 in, 2 out]
                  n3074 = Concatenate Strings(w4098, "=" ("string")) -> (w4099:string)
                  n3075 = local write "S 38"(w4099) -> ()
                }
                frame 38 {
                  n3076 = Match Pattern(string=w4110, regular expression=",") -> (before substring=w4109:string, after substring=w4108:string)  [unwired: 1 in, 2 out]
                  "bs" <- w4109
                  "as" <- w4108
                  n3077 = Concatenate Strings(w4109, w4108) -> (w4105:string)
                  n3078 = property on="Humidity after test 2" class="DigNum (strict)"("Caption.Text"=w4105) -> ()  [unwired: 2 in, 2 out]
                  n3079 = Concatenate Strings(w4105, "=" ("string")) -> (w4107:string)
                  n3080 = property on="Humidity after test" class="DigNum (strict)"("Caption.Text"=w4105) -> ()  [unwired: 2 in, 2 out]
                  n3081 = local write "S 39"(w4107) -> ()
                }
                frame 39 {
                  n3082 = Match Pattern(string=w4117, regular expression=",") -> (before substring=w4116:string, after substring=w4115:string)  [unwired: 1 in, 2 out]
                  "bs" <- w4116
                  "as" <- w4115
                  n3083 = Concatenate Strings(w4116, w4115) -> (w4112:string)
                  n3084 = property on="Temperature before test 2" class="DigNum (strict)"("Caption.Text"=w4112) -> ()  [unwired: 2 in, 2 out]
                  n3085 = property on="Temperature before test" class="DigNum (strict)"("Caption.Text"=w4112) -> ()  [unwired: 2 in, 2 out]
                  n3086 = Concatenate Strings(w4112, "=" ("string")) -> (→"String 34":string)
                }
                frame 40 {
                  n3087 = Match Pattern(string=w4124, regular expression=",") -> (before substring=w4123:string, after substring=w4122:string)  [unwired: 1 in, 2 out]
                  "bs" <- w4123
                  "as" <- w4122
                  n3088 = Concatenate Strings(w4123, w4122) -> (w4119:string)
                  n3089 = property on="Temperature after test 2" class="DigNum (strict)"("Caption.Text"=w4119) -> ()  [unwired: 2 in, 2 out]
                  n3090 = Concatenate Strings(w4119, "=" ("string")) -> (→"String 35":string)
                  n3091 = property on="Temperature after test" class="DigNum (strict)"("Caption.Text"=w4119) -> ()  [unwired: 2 in, 2 out]
                }
                frame 41 {
                  n3092 = property on="AVP" class="DigNum (strict)"("Caption.Text"=w4128) -> ()  [unwired: 2 in, 2 out]
                  n3093 = property on="AVP 2" class="DigNum (strict)"("Caption.Text"=w4128) -> ()  [unwired: 2 in, 2 out]
                  n3094 = Concatenate Strings(w4128, "=" ("string")) -> (→"String 36":string)
                }
                frame 42 {
                  n3095 = property on="MWSD" class="DigNum (strict)"("Caption.Text"=w4131) -> ()  [unwired: 2 in, 2 out]
                  n3096 = property on="MWSD 2" class="DigNum (strict)"("Caption.Text"=w4131) -> ()  [unwired: 2 in, 2 out]
                  n3097 = Concatenate Strings(w4131, "=" ("string")) -> (→"String 37":string)
                }
                frame 43 {
                  n3098 = property on="HCF 2" class="DigNum (strict)"("Caption.Text"=w4134) -> ()  [unwired: 2 in, 2 out]
                  n3099 = property on="HCF" class="DigNum (strict)"("Caption.Text"=w4134) -> ()  [unwired: 2 in, 2 out]
                  n3100 = Concatenate Strings(w4134, "=" ("string")) -> (→"String 38":string)
                }
                frame 44 {
                  n3101 = Concatenate Strings(w4136, "=" ("string")) -> (→"String 39":string)
                  n3102 = property on="WS1.4 2" class="DigNum (strict)"("Caption.Text"=w4136) -> ()  [unwired: 2 in, 2 out]
                  n3103 = property on="WS1.4" class="DigNum (strict)"("Caption.Text"=w4136) -> ()  [unwired: 2 in, 2 out]
                }
                frame 45 {
                  n3104 = property on="Save Results" class="Bool (strict)"("Boolean Text.Text"=w4138) -> ()  [unwired: 2 in, 2 out]
                }
                frame 46 {
                  n3105 = local write "S 47"(w4139) -> ()
                }
                frame 47 {
                  n3106 = local write "S 48"(w4140) -> ()
                }
                frame 48 {
                  n3107 = local write "S 49"(w4141) -> ()
                }
                frame 49 {
                  n3108 = local write "S 50"(w4142) -> ()
                }
                frame 50 {
                  n3109 = local write "S 51"(w4143) -> ()
                }
                frame 51 {
                  n3110 = local write "S 52"(w4144) -> ()
                }
                frame 52 {
                  n3111 = local write "S 53"(w4145) -> ()
                }
                frame 53 {
                  n3112 = local write "S 54"(w4146) -> ()
                }
                frame 54 {
                  n3113 = local write "S 55"(w4147) -> ()
                }
                frame 55 {
                  n3114 = local write "S 56"(w4148) -> ()
                }
                frame 56 {
                  n3115 = local write "S 57"(w4149) -> ()
                }
                frame 57 {
                  n3116 = local write "S 58"(w4150) -> ()
                }
                frame 58 {
